vi "Get Output Value.vi"(10 "Output Values":cluster{"Name":string, "Variant Data":variant}[](array[cluster]), 11 "Step Output in":T1) -> (1 "Found":bool, 2 "Output Value":cluster{"Name":string, "Variant Data":variant}, 3 "Step Output out":T1)   [LabVIEW 2015, in "Execution.lvclass"]
uses:
  Execution.lvclass
  Step/STEP_OUTPUT.ctl
  Step/OUTPUT_DATA_TYPE.ctl
  OutputUI/OUTPUT_CHECK_TYPE.ctl
  Step/OUTPUT_VALUE_TYPE.ctl
  Step.lvclass
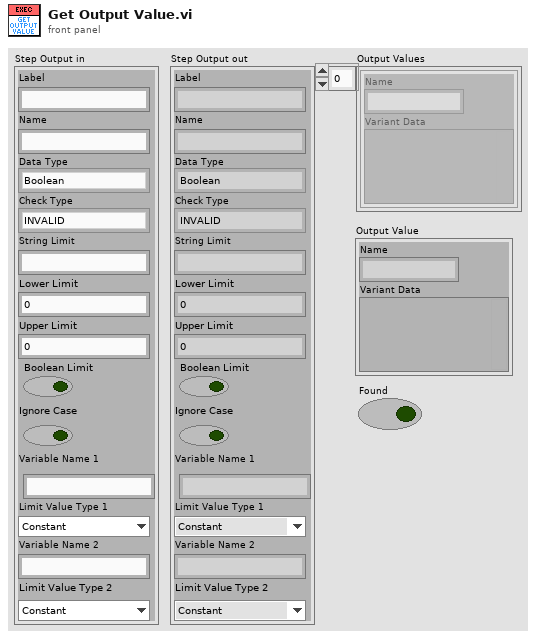
[diagram p1: front panel]
types:
  T1 = typedef "Step.lvclass/STEP_OUTPUT.ctl" = cluster{"Label":string, "Name":string, "Data Type":T2, "Check Type":T3, "String Limit":string, "Lower Limit":dbl, "Upper Limit":dbl, "Boolean Limit":bool, "Ignore Case":bool, "Variable Name 1":string, "Limit Value Type 1":T4, "Variable Name 2":string, "Limit Value Type 2":T4}
  T2 = typedef "Step.lvclass/OUTPUT_DATA_TYPE.ctl" = enum16{"Boolean", "String", "Numeric", "Other"}
  T3 = typedef "Step.lvclass/OUTPUT_CHECK_TYPE.ctl" = enum16{"INVALID", "DO_NOT_CHECK", "RECORD", "VARIABLE", "EQUAL", "NOT_EQUAL", "STR_CONTAINS", "STR_START_WITH", "STR_END_WITH", "STR_REGEX_MATCH", "NUM_GT", "NUM_LT", "NUM_GE", "NUM_LE", "NUM_RANGE", "NUM_RANGE_BDY"}
  T4 = typedef "Step.lvclass/OUTPUT_VALUE_TYPE.ctl" = enum16{"Constant", "Variable"}
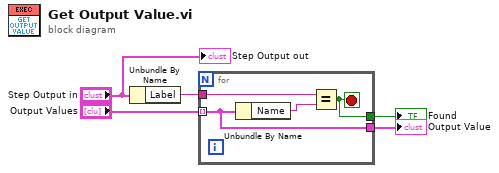
[diagram p0: block diagram]
diagram:
  n1 = Unbundle By Name("Step Output in") -> ("Label"=w3:string)
  n2 = for {
    tunnel: "Output Values" -> [w7] mode=indexing
    tunnel: w3 -> [w8]
    tunnel: [w7] -> w5
    tunnel: [w6] -> w4
    stop <- w6 stop-if-true
    n3 = Unbundle By Name(w7) -> ("Name"=w9:string)
    n4 = Equal?(x=w8, y=w9) -> (x = y?=w6:bool)
  }
  "Output Value" <- w5
  "Found" <- w4
  "Step Output out" <- "Step Output in"
